vi "Motion Profile Call VI.vi"(6 "Synchronication":enum16{"Start", "Wait"}(ring)=enum."Wait", 8 "Command Info In":T1) -> (0 "Command Info Out":T1)   [LabVIEW 2017]
uses:
  <vilib>/Rock Robotics/WPI/Framework/Command Status Info.ctl
  <vilib>/Rock Robotics/WPI/Framework/Completion Status.ctl
  <vilib>/Rock Robotics/WPI/Framework/Completion Notifier.ctl
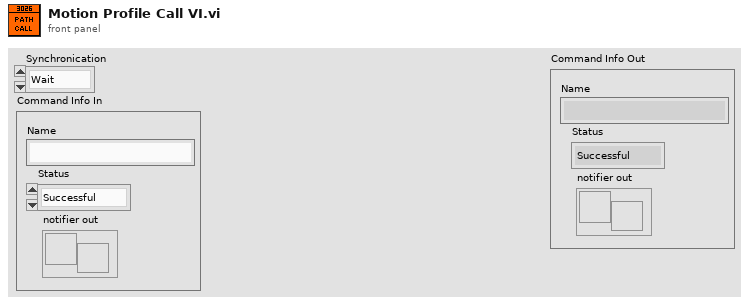
[diagram p1: front panel]
types:
  T1 = typedef "Command Status Info.ctl" = cluster{"Name":string, "Status":T2, "notifier out":T3}
  T2 = typedef "Completion Status.ctl" = enum16{"Successful", "Aborted", "Incomplete"}
  T3 = typedef "Completion Notifier.ctl" = refnum<notifier>
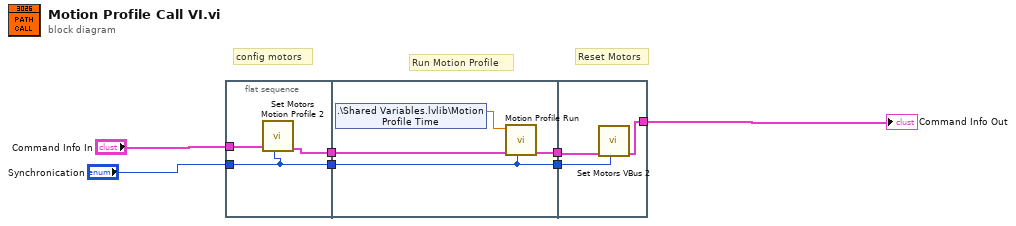
[diagram p0: block diagram]
diagram:
  # "config motors"
  # "Reset Motors"
  # "Run Motion Profile"
  n1 = flat-sequence {
    tunnel: "Command Info In" -> [w9]
    tunnel: "Synchronication" -> [w10]
    tunnel: [w10] -> w3
    tunnel: [w8] -> w2
    tunnel: [w14] -> w4
    tunnel: w3 -> [w12]
    tunnel: w2 -> [w13]
    tunnel: [w12] -> w1
    tunnel: [w15] -> w6
    tunnel: w4 -> [w17]
    tunnel: w1 -> [w16]
    frame #0 {
      n2 = call "Set Motors Motion Profile 2.vi"("Synchronication"=w10, "Command Info In"=w9) -> ("Command Info Out"=w8:T1)  [unwired: 9 in]
    }
    frame #1 {
      n3 = shared-variable ".\\Shared Variables.lvlib\\Motion Profile Time"() -> (w11:dbl)  [unwired: 1 in, 1 out]
      n4 = call "Motion Profile Run.vi"("Synchronication"=w12, "Command Info In"=w13, "Duration"=w11) -> ("Command Info Out"=w14:T1)  [unwired: 8 in]
    }
    frame #2 {
      n5 = call "Set Motors VBus 2.vi"("Synchronication"=w16, "Command Info In"=w17) -> ("Command Info Out"=w15:T1)  [unwired: 9 in]
    }
  }
  "Command Info Out" <- w6
